vi "zad1.vi"() -> ()   [LabVIEW 2017]
panel:
  out "product":i32
  in  "Numeric":i32=10
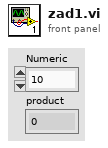
[diagram p1: front panel]
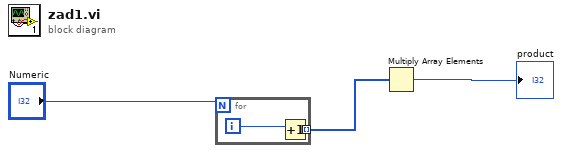
[diagram p0: block diagram]
diagram:
  n1 = for {
    N: "Numeric" -> [_]
    tunnel: [w4] -> w1 mode=indexing
    i -> [w5]
    n2 = Increment(x=w5) -> (x+1=w4:i32)
  }
  n3 = Multiply Array Elements(1:w1) -> (0:→"product":i32)
